vi "Waveform_Delete End Point Attribute.vi"(8 "Error":errorcluster, 11 "Waveform Attributes":variant) -> (0 "Error Out":errorcluster, 3 "Waveform Attributes Out":variant)   [LabVIEW 2024]
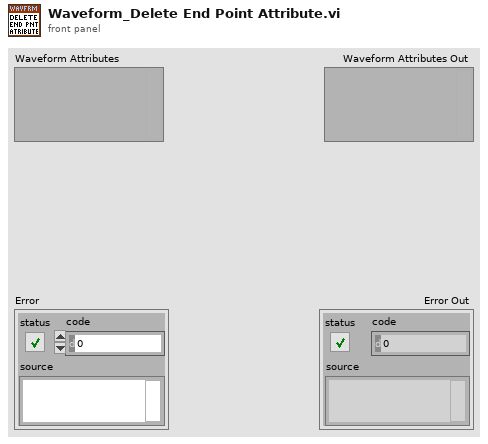
[diagram p1: front panel]
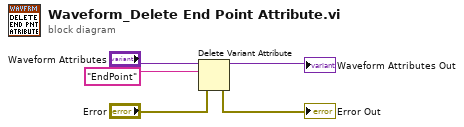
[diagram p0: block diagram]
diagram:
  n1 = Delete Variant Attribute(4:"Error", 6:"EndPoint" ("name"), 7:"Waveform Attributes") -> (0:→"Error Out":errorcluster, 3:→"Waveform Attributes Out":variant)  [unwired: 1 out]
